vi "Stop Core.vi"(6 "final error code":i32, 11 "Websocket Client Handler in":refnum<class "Websocket Client Handler.lvclass">) -> (3 "Websocket Client Handler out":refnum<class "Websocket Client Handler.lvclass">)   [LabVIEW 2016, in "Stream Mediator.lvlib" / "Websocket Client Handler.lvclass"]
doc: "--\nCopyright © 2017 Composed SystemsI All rights reserved.\n\nAuthor: Jon McBee <jon.mcbee@composed.io>\n\nThis library is provided \"AS IS\" ,WITHOUT WARRANTIES OR\nCONDITIONS OF ANY KIND, either express or implied.\n\nComposed Systems -- composed.io\n\nStream 0.0.1.1\nJon McBee - Composed Systems\nCopyright (c) 2017, Composed Systems"
uses:
  <userlib>/Composed Systems/Stream/Mediator/Classes/Websocket Client Handler Actor/Websocket Client Handler/Websocket Client Handler.lvclass
  <userlib>/Composed Systems/Stream/Mediator/Classes/Mediated Asynchronous Actor/Mediated Asynchronous Actor.lvclass
  <vilib>/MediaMongrels Ltd/WebSockets/WebSockets/WebSockets.lvlib
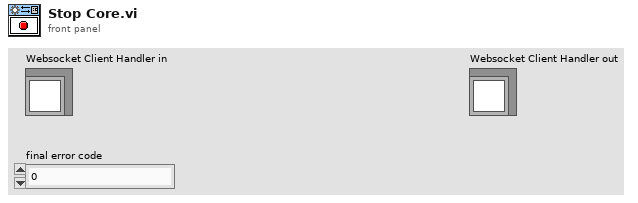
[diagram p1: front panel]
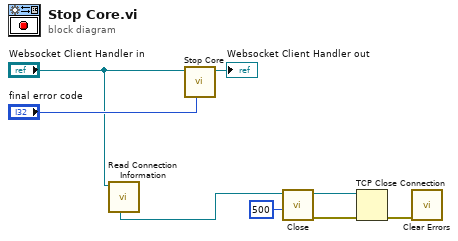
[diagram p0: block diagram]
diagram:
  n1 = call <userlib>:"Read Connection Information.vi"("Websocket Client Handler in"="Websocket Client Handler in") -> ("Connection ID"=w2:refnum<k5>)  [unwired: 8 in, 2 out]
  n2 = call-parent "Stop Core.vi"("final error code"="final error code", "Mediated Asynchronous Actor in"="Websocket Client Handler in") -> ("Mediated Asynchronous Actor out"=→"Websocket Client Handler out":refnum<class "Websocket Client Handler.lvclass">)  [unwired: 9 in]
  n3 = call <vilib>:"Close.vi"("timeout ms (5000)"=500, "WebSocket Connection in"=w2) -> ("error out"=w5:errorcluster, "WebSocket Connection in"=w4:refnum<k5>)  [unwired: 8 in]
  n4 = TCP Close Connection(connection ID=w4, error in (no error)=w5) -> (error out=w6:errorcluster)  [unwired: 1 in, 1 out]
  n5 = call <vilib>:"Clear Errors.vi"("error in (no error)"=w6) -> ()  [unwired: 5 in, 2 out]
